vi "read_master_file.vi"(8 "error in (no error)":errorcluster, 10 "setup file pattern":string[](array[string]), 11 "master file path":path) -> (0 "error out":errorcluster, 3 "setup file paths":string)   [LabVIEW 2017, in "worker.lvlib"]
uses:
  worker.lvlib
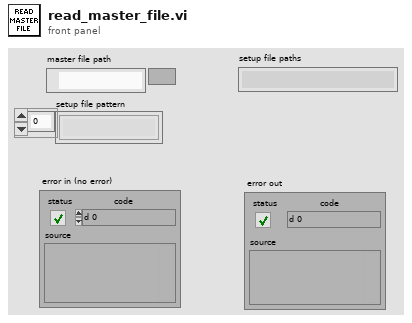
[diagram p1: front panel]
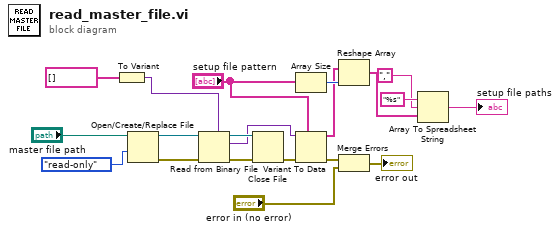
[diagram p0: block diagram]
diagram:
  n1 = To Variant(anything=string[] []) -> (Variant=w1:variant)
  n2 = Open/Create/Replace File(file path (use dialog)="master file path", access (0:read/write)=enum16{"read/write", "read-only", "write-only"}."read-only") -> (refnum out=w18:refnum<file>, error out=w19:errorcluster)  [unwired: 4 in, 1 out]
  n3 = Read from Binary File(5:w1, 8:w19, 11:w18) -> (0:w17:errorcluster, 2:w15:variant, 3:w16:refnum<file>)  [unwired: 3 in, 1 out]
  n4 = Close File(refnum=w16, error in=w17) -> (error out=w11:errorcluster)  [unwired: 1 out]
  n5 = Array Size(array="setup file pattern") -> (size(s)=w14:i32)
  n6 = Variant To Data(error in=w11, type="setup file pattern", Variant=w15) -> (data=w4:string[], error out=w8:errorcluster)
  n7 = Reshape Array(w4, w14) -> (w5:string[])
  n8 = Merge Errors(w8, "error in (no error)") -> (→"error out":errorcluster)
  n9 = Array To Spreadsheet String(delimiter (Tab)=",", array=w5, 3:"%s" ("format string")) -> (spreadsheet string=→"setup file paths":string)
